vi "Read_action.vi"(8 "error in (no error)":errorcluster, 11 "HGF_Configuration in":refnum<class "HGF_Configuration.lvclass">) -> (0 "error out":errorcluster, 2 "All items found?":bool, 3 "HGF_Configuration out":refnum<class "HGF_Configuration.lvclass">)   [LabVIEW 2012, in "HGF_ApplicationBaseClasses.lvlib" / "HGF_Configuration.lvclass"]
uses:
  HGF_Configuration.lvclass
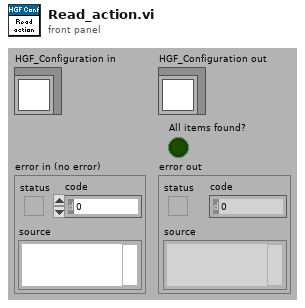
[diagram p1: front panel]
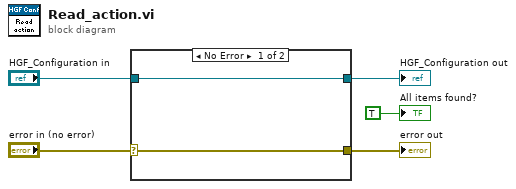
[diagram p0: block diagram]
diagram:
  n1 = case shown="No Error" "error in (no error)" {
    selector: "error in (no error)" -> [w6 w9]
    tunnel: [w6 w9] -> w4
    tunnel: [w7 w8] -> w2
    tunnel: "HGF_Configuration in" -> [w7 w8]
    frame No Error {
    }
    frame Error {
    }
  }
  "error out" <- w4
  "HGF_Configuration out" <- w2
  "All items found?" <- TRUE ("All items found?")
